vi "PH_PowerUnit_BaseClass.PC Shot Action.vi"(0 "i ref in":refnum<vi>, 5 "error in (no error)":errorcluster) -> (14 "i ref out":refnum<vi>, 19 "error out":errorcluster)   [LabVIEW 2014]
doc: "This is the action VI of the Shot event case. It checks the state of the SM and related Devices. If\n\nState SM = \"Wait for Shot Cmd\",\nWaiting Time over? = true,\nState RR = false (closed), \nState PSU = off, \nIgnitron.State Device = on, and\nPPPA PU State = Running,\n\nthen a request state change is send to the SM to get \"Open Ross Relais\"."
uses:
  CSUser/DIMServiceTools/Status.ctl
  PH_PowerUnit_BaseClass.lvlib
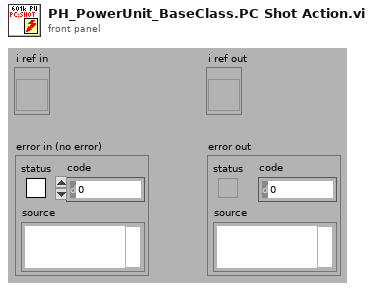
[diagram p1: front panel]
types:
  T1 = typedef "Status.ctl" = i16
  T2 = typedef "PH_PowerUnit_BaseClass.lvlib/PH_PowerUnit_BaseClass.i attribute.ctl" = cluster{"GUI Refs":cluster{"PreAmp enabled":refnum<vi>, "Chiller":refnum<vi>, "PU on":refnum<vi>, "Waiting Time":refnum<vi>, "Delete Inst":refnum<vi>, "Status":refnum<vi>, "Timing":refnum<vi>, "Seq SM State":refnum<vi>}, "Timing Settings":cluster{"Time between Shots [Sec] (30)":dbl, "Waiting Time over?":bool, "Service ID Waiting Time":i32}, "PU in use":bool, "Chiller":cluster{"State Device":T1, "linked?":bool}, "Status":cluster{"Status":T1, "Service ID":i32}, "Timing":cluster{"Instancename":string, "Device Status":T1, "linked?":bool}, "PreAmp Enabling State":T3, "Last Shot":dbl, "Constructor finished":bool, "Sequencer":cluster{"Instance":string, "SM State":string}}
  T3 = typedef "Enabling State.ctl" = i32
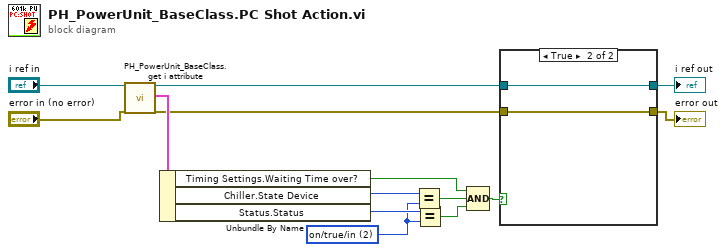
[diagram p0: block diagram]
diagram:
  w7 = T1 2 items=["no info", "off/false/out", "on/true/in", "Failure", "Alarm", "Status 1", "Status 2", "Status 3"] ("Dump Ross Relais.State Device")
  n1 = call "PH_PowerUnit_BaseClass.get i attribute.vi"("i ref in"="i ref in", "error in (no error)"="error in (no error)") -> ("i ref out"=w1:refnum<vi>, "i attribute"=w12:T2, "error out"=w2:errorcluster)  [unwired: 15 in]
  n2 = Unbundle By Name(w12) -> ("Timing Settings.Waiting Time over?"=w6:bool, "Chiller.State Device"=w11:T1, "Status.Status"=w9:T1)
  n3 = Equal?(x=w11, y=w7) -> (x = y?=w10:bool)
  n4 = Equal?(x=w9, y=w7) -> (x = y?=w8:bool)
  n5 = Compound Arithmetic op=AND(w6, w10, w8) -> (w3:bool)
  n6 = case shown="True" w3 {
    tunnel: [w16 w17] -> w13
    tunnel: w1 -> [w15 w18]
    tunnel: w2 -> [w16 w17]
    tunnel: [w15 w18] -> w14
    frame False {
    }
    frame True {
    }
  }
  "i ref out" <- w14
  "error out" <- w13
